vi "SDO byte count ODM.vi"() -> (1 "byte counts":T1)   [LabVIEW 2026, in "MicroPulse_Driver.lvlib"]
uses:
  MicroPulse_Driver.lvlib
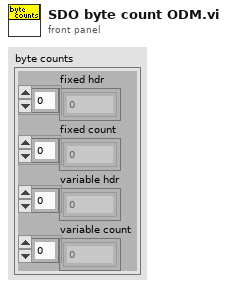
[diagram p1: front panel]
types:
  T1 = cluster{"fixed hdr":u8[], "fixed count":i32[], "variable hdr":u8[], "variable count":i32[]}
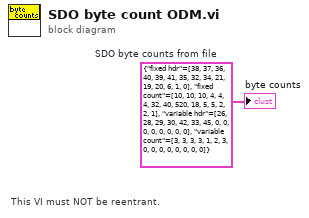
[diagram p0: block diagram]
diagram:
  w1 = T1 {"fixed hdr"=[38, 37, 36, 40, 39, 41, 35, 32, 34, 21, 19, 20, 6, 1, 0], "fixed count"=[10, 10, 10, 4, 4, 4, 32, 40, 520, 18, 5, 5, 2, 2, 1], "variable hdr"=[26, 28, 29, 30, 42, 33, 45, 0, 0, 0, 0, 0, 0, 0, 0], "variable count"=[3, 3, 3, 3, 1, 2, 3, 0, 0, 0, 0, 0, 0, 0, 0]}  # SDO byte counts from file
  # "This VI must NOT be reentrant."
  "byte counts" <- w1
